vi "Write NET_ByteArrayContent.vi"(8 "error in (no error)":errorcluster, 10 "NET_ByteArrayContent":refnum<k24>, 11 "HttpContent_String in":refnum<class "HttpContent_ByteArray.lvclass">) -> (0 "error out":errorcluster, 3 "HttpContent_String out":refnum<class "HttpContent_ByteArray.lvclass">)   [LabVIEW 2018, in "LabVIEWHTTPClient_NET.lvlib" / "HttpContent_ByteArray.lvclass"]
uses:
  HttpContent_ByteArray.lvclass
  C:/Viviota/Projects/R&D/LabVIEW_HTTP_REST_NET/HttpContent/HttpContent.lvclass
  System.Net.Http
  HttpContent/HttpContent.lvclass/HttpContent.ctl
  HttpContent/HttpContent.lvclass
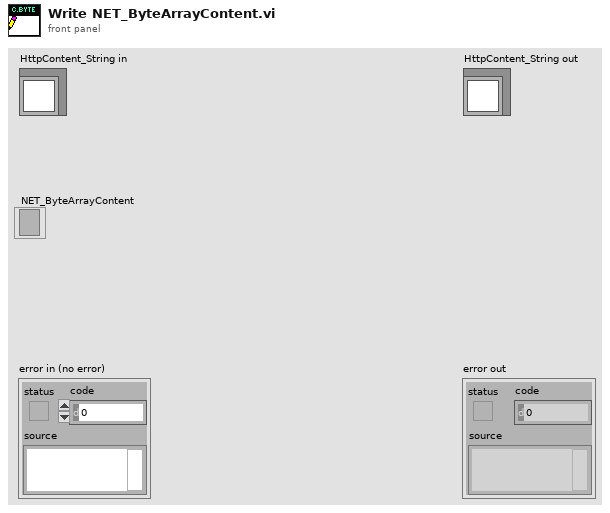
[diagram p1: front panel]
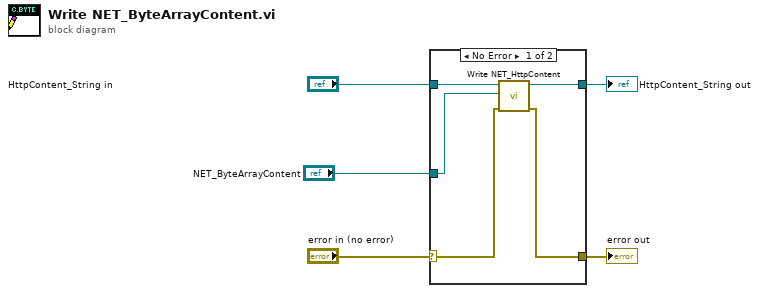
[diagram p0: block diagram]
diagram:
  n1 = case shown="No Error" "error in (no error)" {
    selector: "error in (no error)" -> [w7 w11]
    tunnel: [w8 w11] -> w4
    tunnel: [w9 w12] -> w2
    tunnel: "HttpContent_String in" -> [w10 w12]
    tunnel: "NET_ByteArrayContent" -> [w6 _]
    frame No Error {
      n2 = call "Write NET_HttpContent.vi"("error in (no error)"=w7, "NET_HttpContent"=w6, "HttpContent in"=w10) -> ("error out"=w8:errorcluster, "HttpContent out"=w9:refnum<class "HttpContent_ByteArray.lvclass">)  [unwired: 7 in]
    }
    frame Error {
    }
  }
  "error out" <- w4
  "HttpContent_String out" <- w2
